vi "Options.vi"() -> ()   [LabVIEW 2013, in "main.lvlib"]
uses:
  main.lvlib
  GeneralSettings.vi
  HospitalInfo.vi
  BluetoothSettings.vi
panel:
  in  "optionsCancelBtn":bool caption="CancelBtn"
  in  "optionsOkBtn":bool caption="OkBtn"
  in  "categoryBox":i32(listbox)=5 caption="CategoryBox"
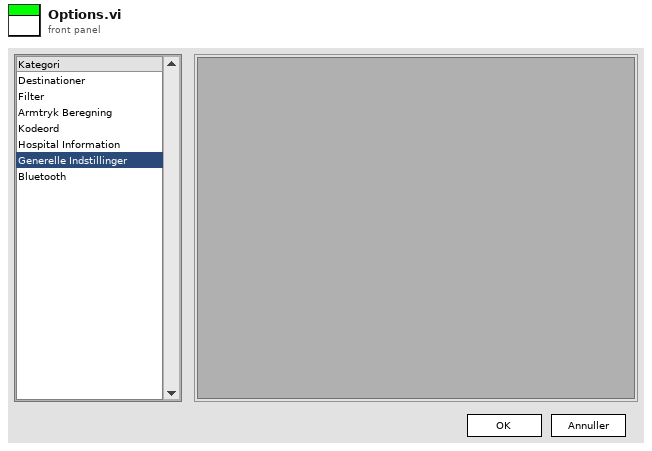
[diagram p1: front panel]
types:
  T1 = cluster{"Loaded":bool, "Name":string, "vi reference":refnum<vi>}
  T2 = cluster{"Loaded":bool, "Name":string, "vi reference":refnum<vi>}[]
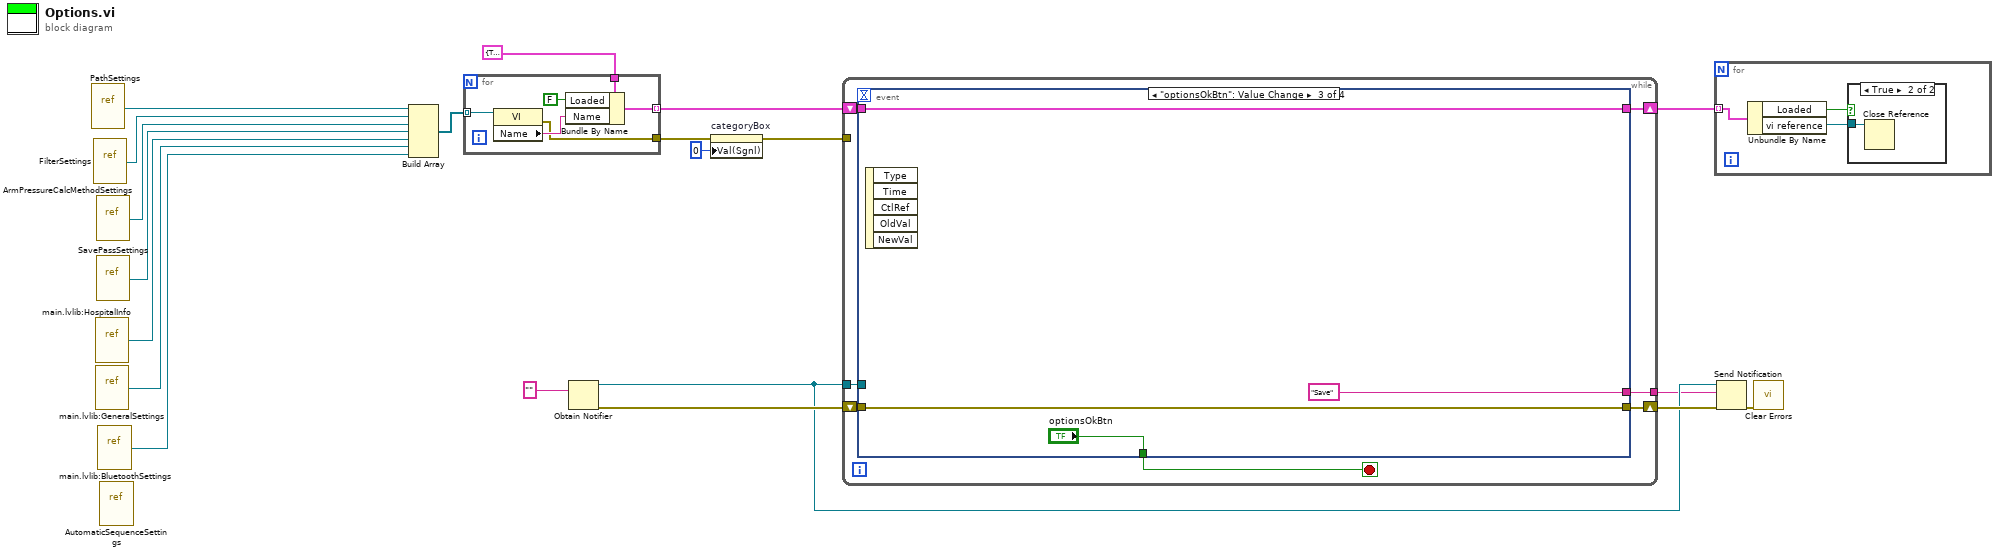
[diagram p0: block diagram]
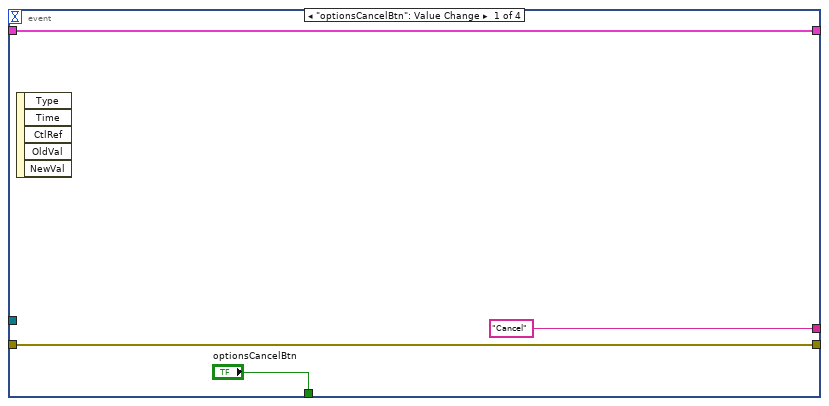
[diagram p3: hidden frame]
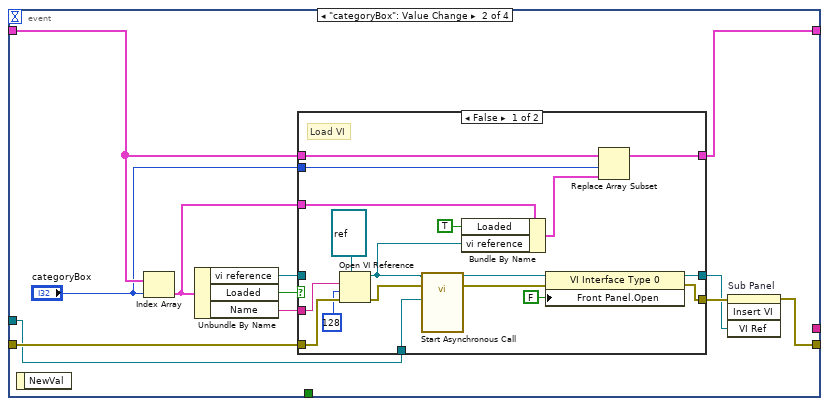
[diagram p4: hidden frame]
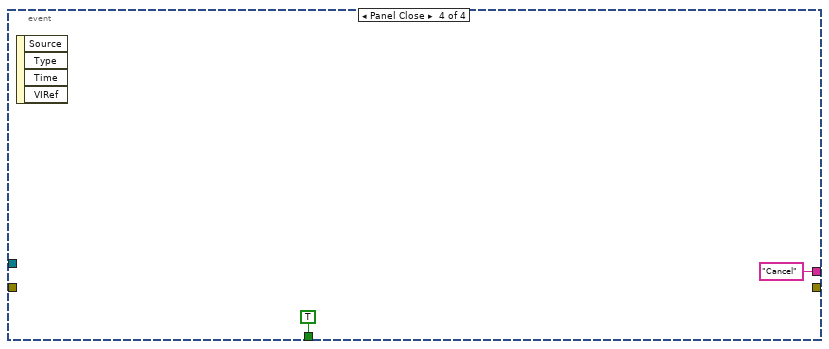
[diagram p6: hidden frame]
diagram:
  n1 = vi-ref "PathSettings.vi"() -> (w16:refnum<vi>)
  n2 = vi-ref "FilterSettings.vi"() -> (w15:refnum<vi>)
  n3 = vi-ref "main.lvlib:HospitalInfo.vi"() -> (w3:refnum<vi>)
  n4 = vi-ref "main.lvlib:GeneralSettings.vi"() -> (w2:refnum<vi>)
  n5 = vi-ref "ArmPressureCalcMethodSettings.vi"() -> (w7:refnum<vi>)
  n6 = vi-ref "SavePassSettings.vi"() -> (w6:refnum<vi>)
  n7 = vi-ref "main.lvlib:BluetoothSettings.vi"() -> (w1:refnum<vi>)
  n8 = vi-ref "AutomaticSequenceSettings.vi"() -> ()  [unwired: 1 out]
  n9 = Build Array(w16, w15, w7, w6, w3, w2, w1) -> (w14:refnum<vi>[])
  n10 = for {
    tunnel: w14 -> [w26] mode=indexing
    tunnel: T1 {"Loaded"=TRUE, "Name"="", "vi reference"=refnum} -> [w25]
    tunnel: [w22] -> w11 mode=indexing
    tunnel: [w21] -> w10
    n11 = property class="VI"(reference=w26) -> (error out=w21:errorcluster, "Name"=w23:string)  [unwired: 1 in, 1 out]
    n12 = Bundle By Name(cluster=w25, "Loaded"=FALSE, "Name"=w23) -> (w22:T1)
  }
  n13 = Obtain Notifier(notification data type="") -> (notifier out=w17:refnum<notifier>, error out=w19:errorcluster)  [unwired: 3 in, 1 out]
  n14 = property on="categoryBox" class="LstBox (strict)"(error in=w10, "Val(Sgnl)"=0 ("Value (Signaling)")) -> (error out=w8:errorcluster)  [unwired: 1 in, 1 out]
  n15 = while {
    tunnel: w17 -> [w32]
    shift-right: [w29] -> w18
    shift-left: w19 -> [w30]
    tunnel: [w28] -> w5
    shift-right: [w27] -> w12
    shift-left: w11 -> [w31]
    tunnel: w8 -> [_]
    stop <- w33 stop-if-true
    n16 = event shown="[2] \"optionsOkBtn\": Value Change" {
      selector: _ -> [_ _ _ _]
      dyn-events: _ -> [_ _ _ _]
      timeout: _ -> [_ _ _ _]
      tunnel: ["optionsCancelBtn" _ "optionsOkBtn" TRUE ("optionsOkBtn")] -> w33
      tunnel: w32 -> [_ w45 _ _]
      tunnel: w31 -> [w35 w41 w71 _]
      tunnel: w30 -> [w34 w49 w73 _]
      tunnel: [w34 w43 w73 _] -> w29
      tunnel: ["Cancel" _ "Save" "Cancel"] -> w28
      tunnel: [w35 w39 w71 _] -> w27
      event "optionsCancelBtn": Value Change {
        n17 = event-data() -> ()  [unwired: 1 in, 5 out]
      }
      event "categoryBox": Value Change {
        n18 = event-data() -> ()  [unwired: 1 in, 1 out]
        n19 = Index Array(array=w41, index="categoryBox") -> (element=w42:T1)
        n20 = Unbundle By Name(w42) -> ("vi reference"=w46:refnum<vi>, "Loaded"=w48:bool, "Name"=w47:string)
        n21 = case shown="False" w48 {
          tunnel: [w55 w68] -> w44
          tunnel: w49 -> [w66 w68]
          tunnel: [w56 w69] -> w38
          tunnel: w47 -> [w65 _]
          tunnel: w46 -> [_ w69]
          tunnel: w45 -> [w52 _]
          tunnel: w42 -> [w64 _]
          tunnel: w41 -> [w62 w70]
          tunnel: "categoryBox" -> [w61 _]
          tunnel: [w59 w70] -> w39
          frame False {
            # "Load VI"
            n22 = Open VI Reference(type specifier VI Refnum (for type only)=refnum<vi> refnum, vi path=w65, options=128, error in (no error)=w66) -> (vi reference=w54:refnum<vi>, error out=w53:errorcluster)  [unwired: 2 in]
            n23 = call-by-ref "Start Asynchronous Call"(reference=w54, error in=w53, "notifier"=w52) -> (reference out=w50:refnum<vi>, error out=w51:errorcluster)  [unwired: 11 in]
            n24 = Bundle By Name(cluster=w64, "Loaded"=TRUE, "vi reference"=w54) -> (w60:T1)
            n25 = property class="VI Interface Type 0"(reference=w50, error in=w51, "Front Panel.Open"=FALSE ("Front Panel Window:Open")) -> (reference out=w56:refnum<vi>, error out=w55:errorcluster)
            n26 = Replace Array Subset(array=w62, new element=w60, index=w61) -> (w59:T2)
          }
          frame True {
          }
        }
        n27 = invoke on="Sub Panel" class="SubPnl" method="Insert VI"(error in=w44, "VI Ref"=w38) -> (error out=w43:errorcluster)  [unwired: 2 in, 3 out]
      }
      event "optionsOkBtn": Value Change {
        n28 = event-data() -> ()  [unwired: 1 in, 5 out]
      }
      event Panel Close {
        n29 = event-data() -> ()  [unwired: 1 in, 4 out]
      }
    }
  }
  n30 = for {
    tunnel: w12 -> [w79] mode=indexing
    n31 = Unbundle By Name(w79) -> ("Loaded"=w78:bool, "vi reference"=w77:refnum<vi>)
    n32 = case shown="True" w78 {
      tunnel: w77 -> [_ w80]
      frame False {
      }
      frame True {
        n33 = Close Reference(reference=w80) -> ()  [unwired: 1 in, 1 out]
      }
    }
  }
  n34 = Send Notification(notification=w5, notifier=w17, error in (no error)=w18) -> (error out=w4:errorcluster)  [unwired: 1 out]
  n35 = call <vilib>:"Clear Errors.vi"("error in (no error)"=w4) -> ()  [unwired: 6 in, 1 out]
